vi "Linear Fit Coefficients PtByPt.vi"(0 "y":dbl format="%0.2f", 1 "x":dbl format="%0.2f", 3 "sample length":i32=100, 4 "initialize":bool) -> (5 "History of x":dbl[](array[numeric]), 6 "History of y":dbl[](array[numeric]), 7 "slope":dbl format="%0.2f", 8 "intercept":dbl format="%0.2f", 10 "error":i32)   [LabVIEW 2020, in "NI_PtbyPt.lvlib"]
doc: "Finds the coefficients <B>slope</B> and <B>intercept</B>, using the least-squares solution, which describe the line that best represents the set of input data points."
uses:
  <vilib>/ptbypt/NI_PtbyPt.lvlib
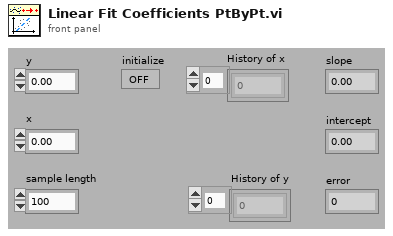
[diagram p1: front panel]
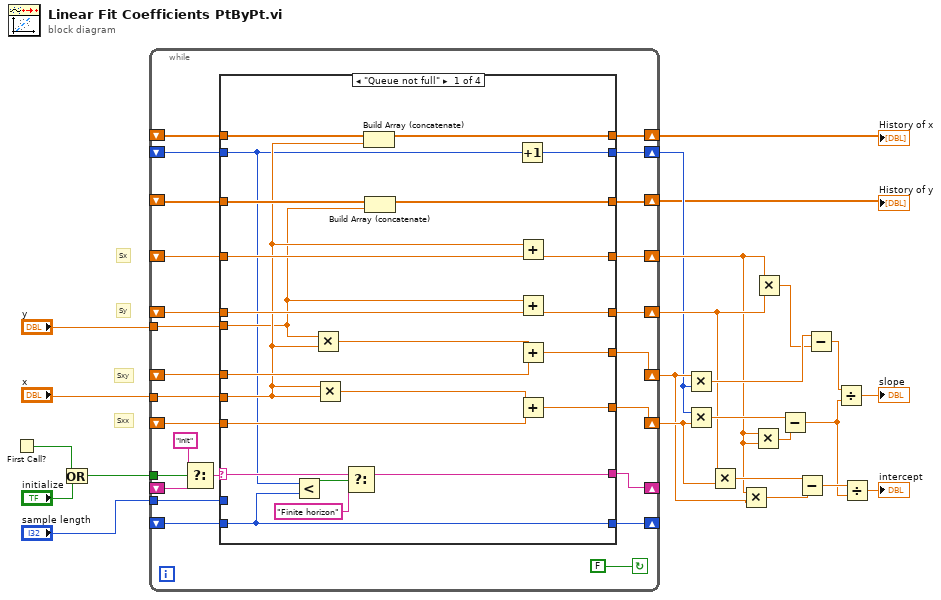
[diagram p0: block diagram]
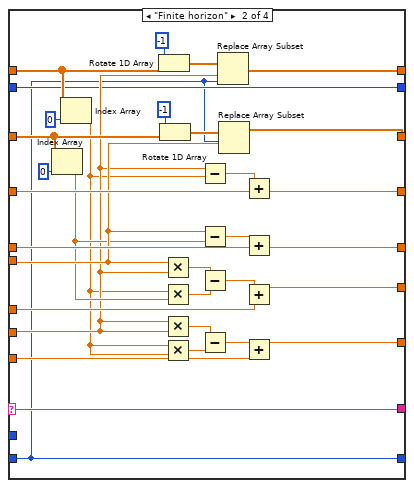
[diagram p2: hidden frame]
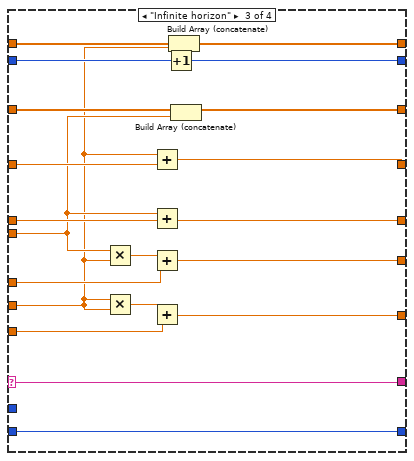
[diagram p3: hidden frame]
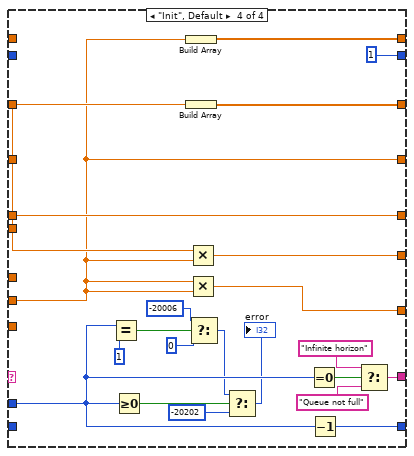
[diagram p4: hidden frame]
diagram:
  # "Sxx"
  # "Sxy"
  # "Sy"
  # "Sx"
  n1 = First Call?() -> (First Call?: T/F=w3:bool)
  n2 = Or(x=w3, y="initialize") -> (x .or. y?=w1:bool)
  n3 = while {
    shift-left: _ -> [w26]
    shift-right: [w31] -> _
    shift-left: _ -> [w32]
    shift-right: [w30] -> _
    tunnel: w1 -> [w33]
    shift-left: _ -> [w37]
    shift-right: [w36] -> w15
    shift-left: _ -> [w38]
    shift-right: [w39] -> w8
    tunnel: "y" -> [w42]
    shift-left: _ -> [w41]
    shift-right: [w40] -> w16
    shift-left: _ -> [w43]
    shift-right: [w44] -> w13
    shift-left: _ -> [w45]
    shift-right: [w28] -> w4
    shift-left: _ -> [w46]
    shift-right: [w27] -> w6
    tunnel: "x" -> [w47]
    tunnel: "sample length" -> [w49]
    shift-left: _ -> [w48]
    shift-right: [w29] -> w5
    stop <- FALSE continue-if-true
    n4 = Select(t="Init", s=w33, f=w32) -> (s? t:f=w35:string)
    n5 = case shown="\"Queue not full\"" w35 {
      selector: w35 -> [w59 w75 w119 _]
      tunnel: w47 -> [w56 w82 w109 w134]
      tunnel: w49 -> [_ _ _ w143]
      tunnel: [w63 w104 w124 w135] -> w29
      tunnel: w48 -> [w64 w99 w125 _]
      tunnel: w46 -> [w50 w74 w123 _]
      tunnel: w45 -> [w62 w97 w121 _]
      tunnel: [w61 w100 w120 w138] -> w28
      tunnel: [w71 w93 w116 w134] -> w44
      tunnel: w43 -> [w72 w94 w117 _]
      tunnel: w42 -> [w55 w89 w111 w139]
      tunnel: w41 -> [w70 w91 w115 _]
      tunnel: [w69 w90 w114 w139] -> w40
      tunnel: [w68 w83 w112 w146] -> w39
      tunnel: w38 -> [w67 w84 w113 _]
      tunnel: w37 -> [w66 w77 w107 _]
      tunnel: [w65 w76 w106 w133] -> w36
      tunnel: [w52 w73 w118 w137] -> w31
      tunnel: [w58 w75 w119 w140] -> w30
      tunnel: [w51 w74 w122 1] -> w27
      tunnel: w26 -> [w52 w73 w118 _]
      frame "Queue not full" {
        n6 = Less?(x=w50, y=w52) -> (x < y?=w60:bool)
        n7 = Multiply(x=w55, y=w56) -> (x*y=w54:dbl)
        n8 = Multiply(x=w56, y=w56) -> (x*y=w53:dbl)
        n9 = Select(t=w59, s=w60, f="Finite horizon") -> (s? t:f=w58:string)
        n10 = Build Array (concatenate)(w64, w56) -> (w63:dbl[])
        n11 = Build Array (concatenate)(w62, w55) -> (w61:dbl[])
        n12 = Increment(x=w50) -> (x+1=w51:i32)
        n13 = Add(x=w56, y=w72) -> (x+y=w71:dbl)
        n14 = Add(x=w55, y=w70) -> (x+y=w69:dbl)
        n15 = Add(x=w54, y=w67) -> (x+y=w68:dbl)
        n16 = Add(x=w53, y=w66) -> (x+y=w65:dbl)
      }
      frame "Finite horizon" {
        n17 = Index Array(array=w97, index=0 ("Index")) -> (element=w88:dbl)
        n18 = Index Array(array=w99, index=0 ("Index")) -> (element=w81:dbl)
        n19 = Rotate 1D Array(1:w99, 2:i16 -1 ("n")) -> (0:w103:dbl[])
        n20 = Rotate 1D Array(1:w97, 2:i16 -1 ("n")) -> (0:w101:dbl[])
        n21 = Multiply(x=w89, y=w82) -> (x*y=w87:dbl)
        n22 = Multiply(x=w81, y=w88) -> (x*y=w86:dbl)
        n23 = Multiply(x=w82, y=w82) -> (x*y=w80:dbl)
        n24 = Multiply(x=w81, y=w81) -> (x*y=w79:dbl)
        n25 = Subtract(x=w82, y=w81) -> (x-y=w95:dbl)
        n26 = Subtract(x=w89, y=w88) -> (x-y=w92:dbl)
        n27 = Subtract(x=w87, y=w86) -> (x-y=w85:dbl)
        n28 = Subtract(x=w80, y=w79) -> (x-y=w78:dbl)
        n29 = Replace Array Subset(array=w103, new element=w82, index=w73) -> (w104:dbl[])
        n30 = Replace Array Subset(array=w101, new element=w89, index=w73) -> (w100:dbl[])
        n31 = Add(x=w95, y=w94) -> (x+y=w93:dbl)
        n32 = Add(x=w92, y=w91) -> (x+y=w90:dbl)
        n33 = Add(x=w85, y=w84) -> (x+y=w83:dbl)
        n34 = Add(x=w78, y=w77) -> (x+y=w76:dbl)
      }
      frame "Infinite horizon" {
        n35 = Multiply(x=w111, y=w109) -> (x*y=w110:dbl)
        n36 = Multiply(x=w109, y=w109) -> (x*y=w108:dbl)
        n37 = Add(x=w109, y=w117) -> (x+y=w116:dbl)
        n38 = Add(x=w111, y=w115) -> (x+y=w114:dbl)
        n39 = Add(x=w110, y=w113) -> (x+y=w112:dbl)
        n40 = Add(x=w108, y=w107) -> (x+y=w106:dbl)
        n41 = Increment(x=w123) -> (x+1=w122:i32)
        n42 = Build Array (concatenate)(w125, w109) -> (w124:dbl[])
        n43 = Build Array (concatenate)(w121, w111) -> (w120:dbl[])
      }
      frame "Init", Default {
        n44 = Equal?(x=w143, y=1) -> (x = y?=w130:bool)
        n45 = Greater Or Equal To 0?(x=w143) -> (x >= 0?=w129:bool)
        n46 = Build Array(w134) -> (w135:dbl[])
        n47 = Build Array(w139) -> (w138:dbl[])
        n48 = Multiply(x=w139, y=w134) -> (x*y=w146:dbl)
        n49 = Multiply(x=w134, y=w134) -> (x*y=w133:dbl)
        n50 = Select(t=-20006 ("f"), s=w130, f=0) -> (s? t:f=w127:i32)
        n51 = Select(t=w127, s=w129, f=-20202) -> (s? t:f=→"error":i32)
        n52 = Equal To 0?(x=w143) -> (x = 0?=w145:bool)
        n53 = Decrement(x=w143) -> (x-1=w137:i32)
        n54 = Select(t="Infinite horizon", s=w145, f="Queue not full") -> (s? t:f=w140:string)
      }
    }
  }
  "History of x" <- w5
  "History of y" <- w4
  n55 = Multiply(x=w8, y=w6) -> (x*y=w22:dbl)
  n56 = Multiply(x=w6, y=w15) -> (x*y=w20:dbl)
  n57 = Multiply(x=w16, y=w15) -> (x*y=w14:dbl)
  n58 = Multiply(x=w13, y=w8) -> (x*y=w12:dbl)
  n59 = Multiply(x=w13, y=w13) -> (x*y=w19:dbl)
  n60 = Multiply(x=w13, y=w16) -> (x*y=w21:dbl)
  n61 = Subtract(x=w20, y=w19) -> (x-y=w10:dbl)
  n62 = Subtract(x=w14, y=w12) -> (x-y=w11:dbl)
  n63 = Subtract(x=w22, y=w21) -> (x-y=w18:dbl)
  n64 = Divide(x=w18, y=w10) -> (x/y=→"slope":dbl)
  n65 = Divide(x=w11, y=w10) -> (x/y=→"intercept":dbl)
